vi "TCP Write.vi"(11 "Message Queues out":T1) -> ()   [LabVIEW 2018, in "TCP Library.lvlib"]
uses:
  Lauda Integral XT-150 TCU/TCP Library.lvlib
  Main/Main Queue Cluster.ctl
  support/Message Queue/Message Cluster.ctl
  TCP Multiple Connections State.ctl
  Tag VIs/Tag FGV Operation Enum.ctl
  support/Message Queue/Enqueue Message (Single).vi
  <vilib>/addons/_JKI.lib/Serialization/JSON/JKI JSON Serialization.lvlib
  Shared Variables/Dynamic Shared Variables.lvlib
  support/Message Queue/Message Queue.lvlib
panel:
  in  "error in (no error)":errorcluster
  in  "address":string="10.131.72.83"
  in  "port":u16=50023
  out "decimal integer string":string
  out "length":i32
  out "*(type *) &x":string
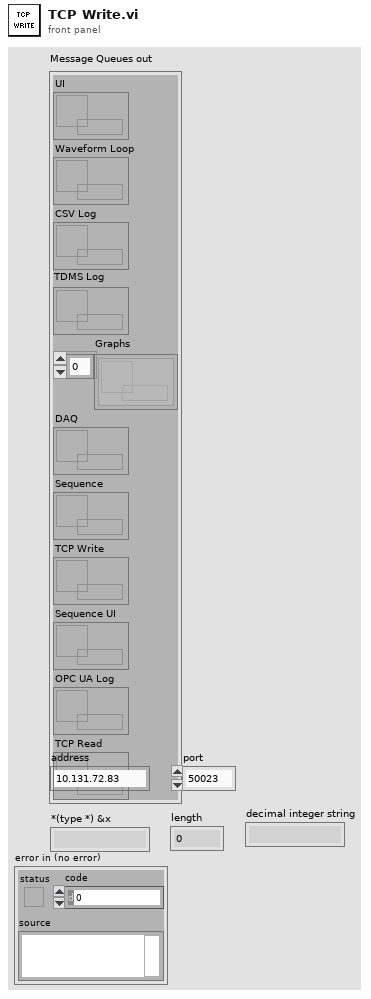
[diagram p1: front panel]
types:
  T1 = typedef "Main Queue Cluster.ctl" = cluster{"UI":refnum<queue>, "Waveform Loop":refnum<queue>, "CSV Log":refnum<queue>, "TDMS Log":refnum<queue>, "Graphs":refnum<queue>[], "DAQ":refnum<queue>, "Sequence":refnum<queue>, "TCP Write":refnum<queue>, "Sequence UI":refnum<queue>, "OPC UA Log":refnum<queue>, "TCP Read":refnum<queue>}
  T2 = typedef "TCP Library.lvlib/TCP Multiple Connections State.ctl" = enum16{"Initialize", "Status Check", "Send Data", "Stop"}
  T3 = cluster{"listener ID":refnum<k5>, "State":T2, "Clients":refnum<k5>[], "ELN Number":string}
  T4 = typedef "Tag FGV Operation Enum.ctl" = enum16{"Init", "Set Notification Queue", "Create Tag", "Commit", "Write Tag (Numeric)", "Write Tag (Boolean)", "Read All Tags", "Read One Tag", "Delete Tag Category", "Set Alarm Parameters (Numeric)", "Set Alarm Parameters (Boolean)", "Enable All Alarms", "Disable All Alarms", "Delete All Tags", "Read Alarms", "Ack Alarm"}
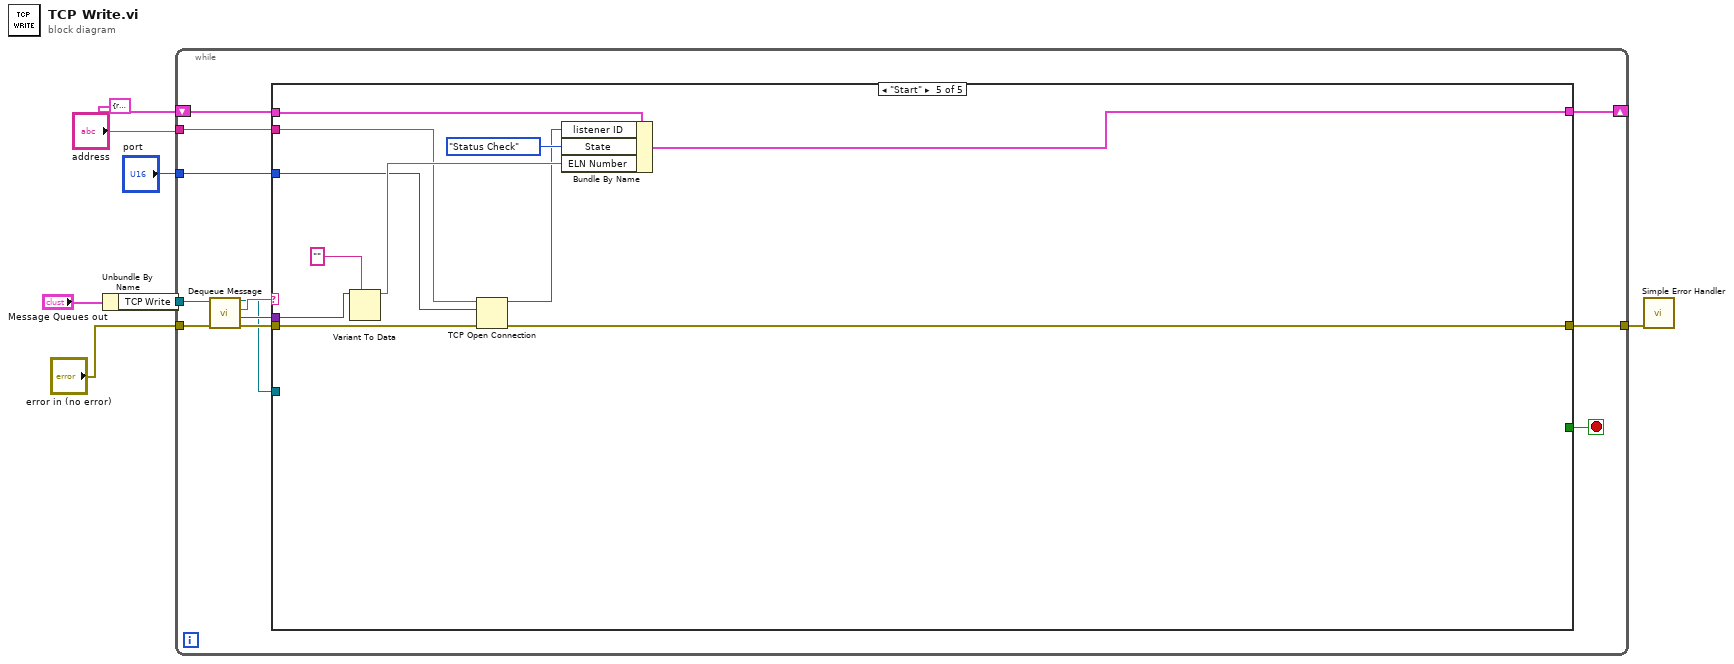
[diagram p0: block diagram]
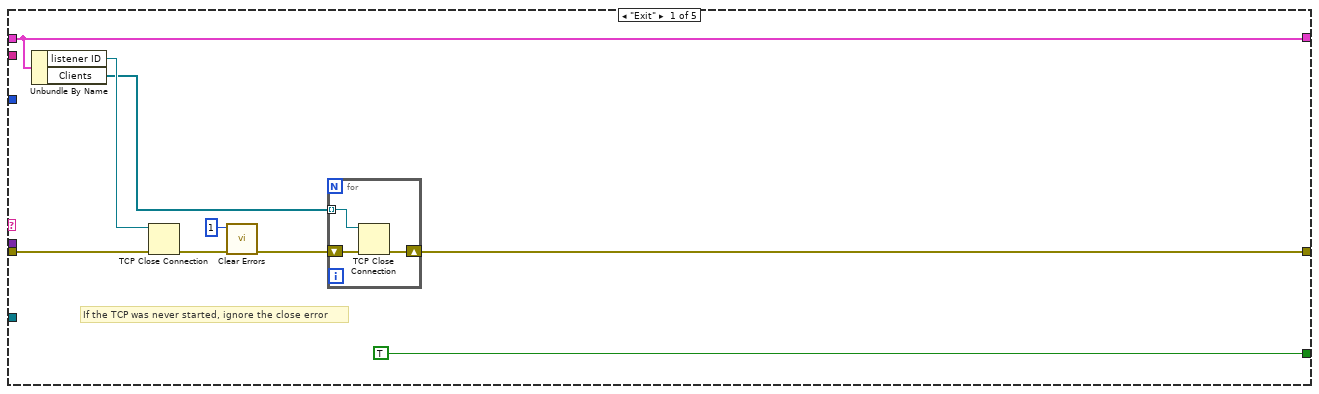
[diagram p2: hidden frame]
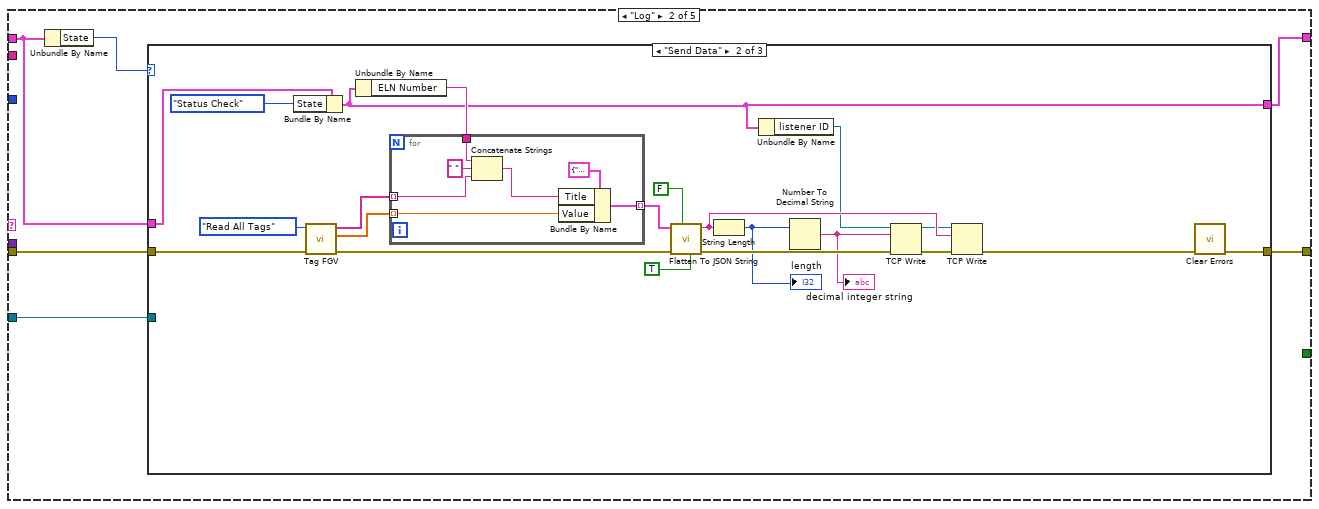
[diagram p3: hidden frame]
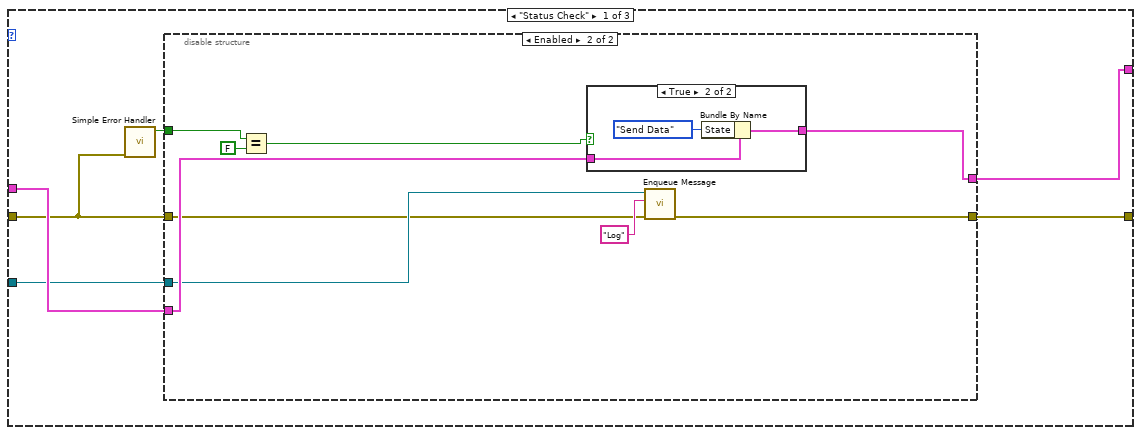
[diagram p4: hidden frame]
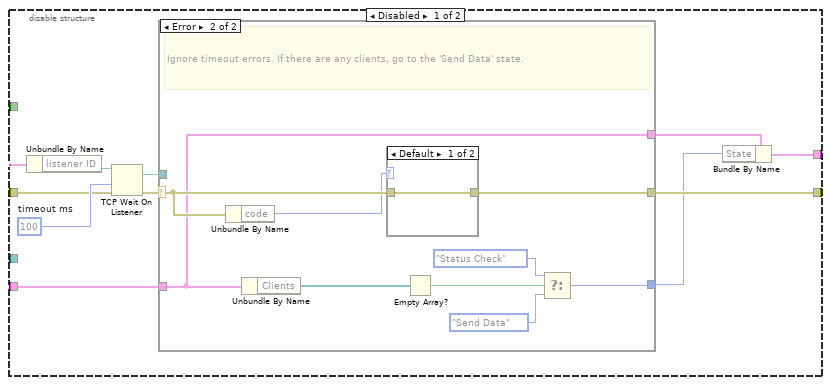
[diagram p5: hidden frame]
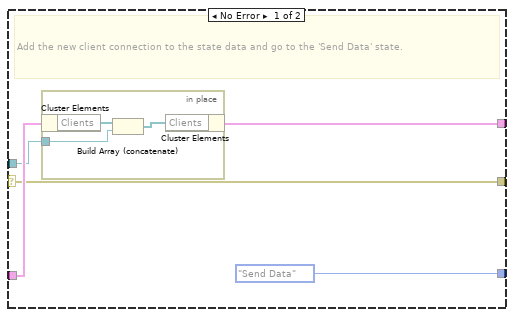
[diagram p6: hidden frame]
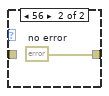
[diagram p7: hidden frame]
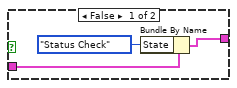
[diagram p8: hidden frame]
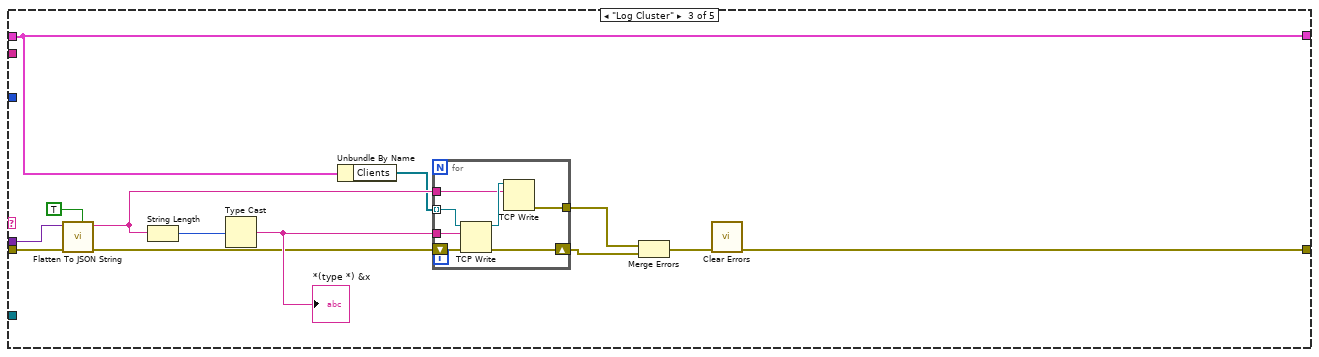
[diagram p10: hidden frame]
diagram:
  n1 = Unbundle By Name("Message Queues out") -> ("TCP Write"=w6:refnum<queue>)
  n2 = while {
    tunnel: w6 -> [w17]
    shift-right: [w14] -> _
    shift-left: T3 {"listener ID"=refnum, "State"=enum."Initialize", "Clients"=[], "ELN Number"=""} -> [w13]
    tunnel: [w12] -> w4
    tunnel: "port" -> [w11]
    tunnel: "address" -> [w10]
    tunnel: "error in (no error)" -> [w9]
    stop <- w16 stop-if-true
    n3 = call "Dequeue Message.vi"("error in (no error)"=w9, "Message Queue"=w17) -> ("error out"=w18:errorcluster, "Message Data"=w15:variant, "Message"=w19:string, "dup Message Queue"=w8:refnum<queue>)  [unwired: 6 in]
    n4 = case shown="\"Start\"" w19 {
      tunnel: w18 -> [w28 w37 w122 w138 w141]
      tunnel: [TRUE _ _ _ _] -> w16
      tunnel: w15 -> [_ _ w121 _ w147]
      tunnel: [w23 w34 w118 w139 w149] -> w14
      tunnel: w13 -> [w23 w35 w118 w139 w150]
      tunnel: [w24 w33 w120 w138 w140] -> w12
      tunnel: w11 -> [_ _ _ _ w143]
      tunnel: w10 -> [_ _ _ _ w142]
      tunnel: w8 -> [_ w32 _ _ _]
      frame "Exit" {
        # "If the TCP was never started, ignore the close error"
        n5 = Unbundle By Name(w23) -> ("listener ID"=w26:refnum<k5>, "Clients"=w25:refnum<k5>[])
        n6 = TCP Close Connection(connection ID=w26, error in (no error)=w28) -> (error out=w22:errorcluster)  [unwired: 1 in, 1 out]
        n7 = call <vilib>:"Clear Errors.vi"("error in (no error)"=w22, "specific error code to clear (0: all)"=1) -> ("error out"=w21:errorcluster)  [unwired: 4 in, 1 out]
        n8 = for {
          shift-right: [w30] -> w24
          shift-left: w21 -> [w31]
          tunnel: w25 -> [w29] mode=indexing
          n9 = TCP Close Connection(connection ID=w29, error in (no error)=w31) -> (error out=w30:errorcluster)  [unwired: 1 in, 1 out]
        }
      }
      frame "Log" {
        n10 = Unbundle By Name(w35) -> ("State"=w36:T2)
        n11 = case shown="\"Send Data\"" w36 {
          tunnel: w37 -> [w40 w108 w116]
          tunnel: w35 -> [w43 w99 w117]
          tunnel: [w41 w92 w117] -> w34
          tunnel: [w42 w97 w116] -> w33
          tunnel: w32 -> [w38 _ _]
          frame "Status Check" {
            n12 = call <vilib>:"Simple Error Handler.vi"("error in (no error)"=w40) -> ("error?"=w39:bool)  [unwired: 4 in, 4 out]
            n13 = disable-structure shown="Enabled" {
              disable-tunnel: w43 -> [w53 w79]
              disable-tunnel: [w52 w73] -> w42
              disable-tunnel: [w45 w78] -> w41
              disable-tunnel: w40 -> [w44 w74]
              disable-tunnel: w39 -> [_ w80]
              disable-tunnel: w38 -> [_ w76]
              frame Disabled {
                w51 = 100  # timeout ms
                n14 = Unbundle By Name(w53) -> ("listener ID"=w48:refnum<k5>)
                n15 = TCP Wait On Listener(8:w44, 9:w51, 11:w48) -> (0:w50:errorcluster, 4:w49:refnum<k5>)  [unwired: 4 out]
                n16 = case shown="Error" w50 {
                  selector: w50 -> [w56 w70]
                  tunnel: [TCP_Multiple_Connections_State."Send Data" ("States") w64] -> w46
                  tunnel: w49 -> [w57 _]
                  tunnel: w53 -> [w58 w67]
                  tunnel: [w55 w67] -> w47
                  tunnel: [w56 w68] -> w52
                  frame No Error {
                    # "Add the new client connection to the state data and go to the 'Send Data' state."
                    n17 = in-place {
                      in-place-border: w57 -> [w59]
                      n18 = in-place-cluster #1(w58) -> ("Clients"=w61:refnum<k5>[])
                      n19 = Build Array (concatenate)(w61, w59) -> (w60:refnum<k5>[])
                      n20 = in-place-cluster #1("Clients"=w60) -> (w55:T3)
                    }
                  }
                  frame Error {
                    # "Ignore timeout errors. If there are any clients, go to the 'Send Data' state."
                    n21 = Unbundle By Name(w70) -> ("code"=w69:i32)
                    n22 = Unbundle By Name(w67) -> ("Clients"=w66:refnum<k5>[])
                    n23 = case shown="Default" w69 {
                      tunnel: w70 -> [w71 _]
                      tunnel: [w71 w72] -> w68
                      frame Default {
                      }
                      frame 56 {
                        w72 = errorcluster {"status"=FALSE, "code"=0, "source"=""}  # no error
                      }
                    }
                    n24 = Empty Array?(array=w66) -> (empty?=w65:bool)
                    n25 = Select(t=TCP_Multiple_Connections_State."Status Check" ("States"), s=w65, f=TCP_Multiple_Connections_State."Send Data" ("States")) -> (s? t:f=w64:T2)
                  }
                }
                n26 = Bundle By Name(cluster=w47, "State"=w46) -> (w45:T3)
              }
              frame Enabled {
                n27 = Equal?(x=w80, y=FALSE) -> (x = y?=w77:bool)
                n28 = case shown="True" w77 {
                  tunnel: w79 -> [w82 w87]
                  tunnel: [w83 w86] -> w78
                  frame False {
                    n29 = Bundle By Name(cluster=w82, "State"=TCP_Multiple_Connections_State."Status Check") -> (w83:T3)
                  }
                  frame True {
                    n30 = Bundle By Name(cluster=w87, "State"=TCP_Multiple_Connections_State."Send Data") -> (w86:T3)
                  }
                }
                n31 = call-poly "Enqueue Message.vi"("error in (no error)"=w74, "Message"="Log", "Message Queue"=w76) -> ("error out"=w73:errorcluster)  [unwired: 7 in, 1 out]
              }
            }
          }
          frame "Send Data" {
            n32 = Bundle By Name(cluster=w99, "State"=TCP_Multiple_Connections_State."Status Check" ("Initial State")) -> (w92:T3)
            n33 = call "Tag FGV.vi"("error in (no error)"=w108, "Operation"=Tag_FGV_Operation_Enum."Read All Tags") -> ("error out"=w101:errorcluster, "Tag Values"=w103:dbl[], "Tag Names"=w104:string[])  [unwired: 4 in, 3 out]
            n34 = Unbundle By Name(w92) -> ("ELN Number"=w96:string)
            n35 = for {
              tunnel: w104 -> [w112] mode=indexing
              tunnel: w103 -> [w114] mode=indexing
              tunnel: [w113] -> w102 mode=indexing
              tunnel: w96 -> [w110]
              n36 = Concatenate Strings(w110, " " ("string"), w112) -> (w111:string)
              n37 = Bundle By Name(cluster=cluster{"Title":string, "Value":dbl} {"Title"="", "Value"=0.0}, "Title"=w111, "Value"=w114) -> (w113:cluster{"Title":string, "Value":dbl})
            }
            n38 = call <vilib>:"Flatten To JSON String.vi"("Enums As String (F)"=TRUE, "Multiline (T)"=FALSE, "error in (no error)"=w101, "Variant"=w102) -> ("error out"=w100:errorcluster, "JSON String"=w107:string)  [unwired: 6 in]
            n39 = String Length(string=w107) -> (length=w95:i32)
            "length" <- w95
            n40 = Unbundle By Name(w92) -> ("listener ID"=w91:refnum<k5>)
            n41 = Number To Decimal String(number=w95) -> (decimal integer string=w94:string)  [unwired: 1 in]
            "decimal integer string" <- w94
            n42 = TCP Write(connection ID=w91, data in=w94, error in (no error)=w100) -> (connection ID out=w93:refnum<k5>, error out=w90:errorcluster)  [unwired: 2 out]
            n43 = TCP Write(connection ID=w93, data in=w107, error in (no error)=w90) -> (error out=w89:errorcluster)  [unwired: 3 out]
            n44 = call <vilib>:"Clear Errors.vi"("error in (no error)"=w89) -> ("error out"=w97:errorcluster)  [unwired: 5 in, 1 out]
          }
          frame Default {
          }
        }
      }
      frame "Log Cluster" {
        n45 = call <vilib>:"Flatten To JSON String.vi"("Enums As String (F)"=TRUE, "error in (no error)"=w122, "Variant"=w121) -> ("error out"=w123:errorcluster, "JSON String"=w127:string)  [unwired: 7 in]
        n46 = String Length(string=w127) -> (length=w129:i32)
        n47 = Type Cast(x=w129) -> (*(type *) &x=w128:string)  [unwired: 1 out]
        "*(type *) &x" <- w128
        n48 = Unbundle By Name(w118) -> ("Clients"=w119:refnum<k5>[])
        n49 = for {
          tunnel: w128 -> [w136]
          tunnel: w127 -> [w135]
          tunnel: [w134] -> w125
          shift-right: [w133] -> w124
          shift-left: w123 -> [w132]
          tunnel: w119 -> [w131] mode=indexing
          n50 = TCP Write(connection ID=w131, data in=w136, error in (no error)=w132) -> (connection ID out=w137:refnum<k5>, error out=w133:errorcluster)  [unwired: 2 out]
          n51 = TCP Write(connection ID=w137, data in=w135) -> (error out=w134:errorcluster)  [unwired: 1 in, 3 out]
        }
        n52 = Merge Errors(w125, w124) -> (w126:errorcluster)
        n53 = call <vilib>:"Clear Errors.vi"("error in (no error)"=w126) -> ("error out"=w120:errorcluster)  [unwired: 5 in, 1 out]
      }
      frame Default {
      }
      frame "Start" {
        n54 = Variant To Data(type="", Variant=w147) -> (data=w145:string)  [unwired: 1 in, 1 out]
        n55 = TCP Open Connection(address=w142, remote port or service name=w143, error in (no error)=w141) -> (connection ID=w144:refnum<k5>, error out=w140:errorcluster)  [unwired: 2 in]
        n56 = Bundle By Name(cluster=w150, "listener ID"=w144, "State"=TCP_Multiple_Connections_State."Status Check" ("Initial State"), "ELN Number"=w145) -> (w149:T3)
      }
    }
  }
  n57 = call <vilib>:"Simple Error Handler.vi"("error in (no error)"=w4) -> ()  [unwired: 4 in, 5 out]
